vi "CreateFileFlowDataEvent.vi"(8 "error in (no error)":errorcluster, 9 "data event":T5, 10 "data event config":T15, 11 "data flow":T1) -> (0 "error out":errorcluster, 1 "data event ref":T13)   [LabVIEW 2017, in "CmsDataEventCreator.lvlib"]
uses:
  <vilib>/addons/InsightCM/Devices/Shared/Cms/CmsDataEventCreator/CmsDataEventCreator.lvlib
  <vilib>/addons/InsightCM/Devices/Shared/Cms/CmsDataEventCreator/controls/DataEventConfig.ctl
  <vilib>/addons/InsightCM/Devices/Shared/Cms/CmsDataEventCreator/controls/AcqParams.ctl
  <vilib>/addons/InsightCM/Devices/Shared/Common/DataAccumulator/controls/AccumulationSettings.ctl
  <vilib>/addons/InsightCM/Devices/Shared/Common/DataAccumulator/controls/accumulationType.ctl
  <vilib>/addons/InsightCM/Devices/Shared/Common/DVRBuffer/controls/BufferLocation.ctl
  <vilib>/addons/PointValueMap/controls/PointMap.ctl
  <vilib>/addons/InsightCM/Devices/Shared/Common/FileFlow/controls/data_eventRef.ctl
  <vilib>/addons/InsightCM/Devices/Shared/Common/DataEvent/controls/EventReference.ctl
  <vilib>/addons/InsightCM/Devices/Shared/Common/DataEvent/controls/Event.ctl
  <vilib>/addons/InsightCM/MessageBus/Base/controls/DataEvent.ctl
  <vilib>/addons/InsightCM/MessageBus/Base/controls/KeyValuePair.ctl
  <vilib>/addons/InsightCM/Devices/Shared/Common/DataEvent/controls/DataSet.ctl
  <vilib>/addons/InsightCM/MessageBus/Base/controls/DataSetMetadata.ctl
  <vilib>/addons/InsightCM/MessageBus/Base/controls/TrendPoint.ctl
  <vilib>/addons/InsightCM/MessageBus/Base/controls/TrendAlarmUpdate.ctl
  <vilib>/addons/InsightCM/MessageBus/Base/controls/TrendAlarmTransition.ctl
  <vilib>/addons/InsightCM/Devices/Shared/Common/DataFlow/controls/Data.ctl
  <vilib>/addons/InsightCM/Utilities/DataAccessors/controls/wfmSGL_DVR.ctl
  <vilib>/addons/InsightCM/Devices/Shared/Common/DataFlow/controls/Type.ctl
  <vilib>/addons/PointValueMap/PointValueMap.lvlib
  <vilib>/addons/InsightCM/Devices/Shared/Common/DataEvent/DataEvent.lvlib
  <vilib>/addons/InsightCM/Devices/Shared/Common/FileFlow/FileFlow.lvlib
  <vilib>/addons/InsightCM/Devices/Shared/Common/DataFlow/DataFlow.lvlib
  <vilib>/addons/InsightCM/Devices/Shared/Common/DataAccumulator/DataAccumulator.lvlib
  <vilib>/addons/InsightCM/Devices/Shared/Common/DVRBuffer/DVRBuffer.lvlib
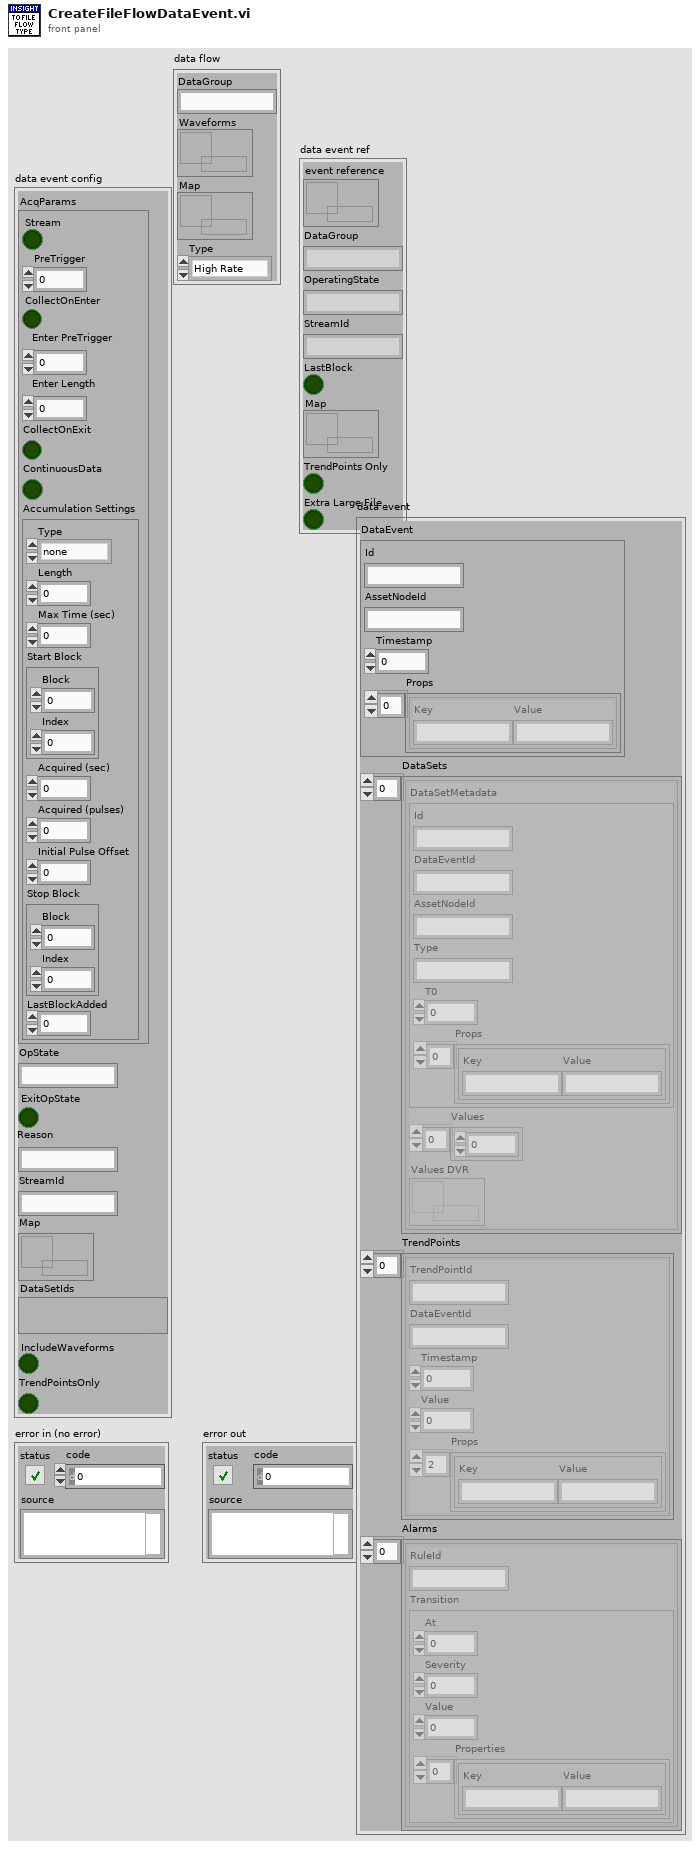
[diagram p1: front panel]
types:
  T1 = typedef "DataFlow.lvlib/Data.ctl" = cluster{"DataGroup":string, "Waveforms":T2, "Map":T3, "Type":T4}
  T2 = typedef "wfmSGL_DVR.ctl" = refnum<data-value>
  T3 = typedef "PointValueMap.lvlib/PointMap.ctl" = refnum<data-value>
  T4 = typedef "DataFlow.lvlib/Type.ctl" = enum16{"High Rate", "Low Rate", "Burst Mode"}
  T5 = typedef "DataEvent.lvlib/Event.ctl" = cluster{"DataEvent":T6, "DataSets":T8[], "TrendPoints":T10[], "Alarms":T11[]}
  T6 = typedef "DataEvent.ctl" = cluster{"Id":string, "AssetNodeId":string, "Timestamp":i64, "Props":T7[]}
  T7 = typedef "KeyValuePair.ctl" = cluster{"Key":string, "Value":string}
  T8 = typedef "DataEvent.lvlib/DataSet.ctl" = cluster{"DataSetMetadata":T9, "Values":sgl[], "Values DVR":refnum<data-value>}
  T9 = typedef "DataSetMetadata.ctl" = cluster{"Id":string, "DataEventId":string, "AssetNodeId":string, "Type":string, "T0":i64, "Props":T7[]}
  T10 = typedef "TrendPoint.ctl" = cluster{"TrendPointId":string, "DataEventId":string, "Timestamp":i64, "Value":dbl, "Props":T7[]}
  T11 = typedef "TrendAlarmUpdate.ctl" = cluster{"RuleId":string, "Transition":T12}
  T12 = typedef "TrendAlarmTransition.ctl" = cluster{"At":i64, "Severity":i32, "Value":dbl, "Properties":T7[]}
  T13 = typedef "FileFlow.lvlib/data_eventRef.ctl" = cluster{"event reference":T14, "DataGroup":string, "OperatingState":string, "StreamId":string, "LastBlock":bool, "Map":T3, "TrendPoints Only":bool, "Extra Large File":bool}
  T14 = typedef "DataEvent.lvlib/EventReference.ctl" = refnum<data-value>
  T15 = typedef "CmsDataEventCreator.lvlib/DataEventConfig.ctl" = cluster{"AcqParams":T16, "OpState":string, "ExitOpState":bool, "Reason":string, "StreamId":string, "Map":T3, "DataSetIds":variant, "IncludeWaveforms":bool, "TrendPointsOnly":bool}
  T16 = typedef "CmsDataEventCreator.lvlib/AcqParams.ctl" = cluster{"Stream":bool, "PreTrigger":i32, "CollectOnEnter":bool, "Enter PreTrigger":i32, "Enter Length":dbl, "CollectOnExit":bool, "ContinuousData":bool, "Accumulation Settings":T17}
  T17 = typedef "DataAccumulator.lvlib/AccumulationSettings.ctl" = cluster{"Type":T18, "Length":dbl, "Max Time (sec)":dbl, "Start Block":T19, "Acquired (sec)":dbl, "Acquired (pulses)":i32, "Initial Pulse Offset":dbl, "Stop Block":T19, "LastBlockAdded":u32}
  T18 = typedef "DataAccumulator.lvlib/accumulationType.ctl" = enum16{"none", "seconds", "revolutions"}
  T19 = typedef "DVRBuffer.lvlib/BufferLocation.ctl" = cluster{"Block":u32, "Index":i32}
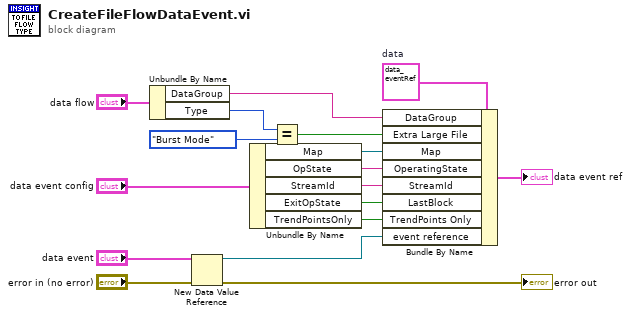
[diagram p0: block diagram]
diagram:
  w11 = T13 {"event reference"=refnum, "DataGroup"="", "OperatingState"="", "StreamId"="", "LastBlock"=FALSE, "Map"=refnum, "TrendPoints Only"=FALSE, "Extra Large File"=FALSE}  # data
  n1 = Unbundle By Name("data flow") -> ("DataGroup"=w4:string, "Type"=w3:T4)
  n2 = New Data Value Reference(data value="data event", error in="error in (no error)") -> (data value reference=w6:refnum<data-value>, error out=→"error out":errorcluster)
  n3 = Unbundle By Name("data event config") -> ("Map"=w12:T3, "OpState"=w15:string, "StreamId"=w14:string, "ExitOpState"=w13:bool, "TrendPointsOnly"=w10:bool)
  n4 = Equal?(x=w3, y=Type."Burst Mode") -> (x = y?=w1:bool)
  n5 = Bundle By Name(cluster=w11, "DataGroup"=w4, "Extra Large File"=w1, "Map"=w12, "OperatingState"=w15, "StreamId"=w14, "LastBlock"=w13, "TrendPoints Only"=w10, "event reference"=w6) -> (→"data event ref":T13)
